vi "AssertControlValueByPath.vi"(0 "VI Reference In":refnum<vi>, 5 "Control Path":string[](array[string]), 11 "error in":errorcluster) -> (4 "VI Reference Out":refnum<vi>, 6 "Value":variant, 15 "error out":errorcluster)   [LabVIEW 2016]
doc: "This VI sets the value of top level controls in other VI"
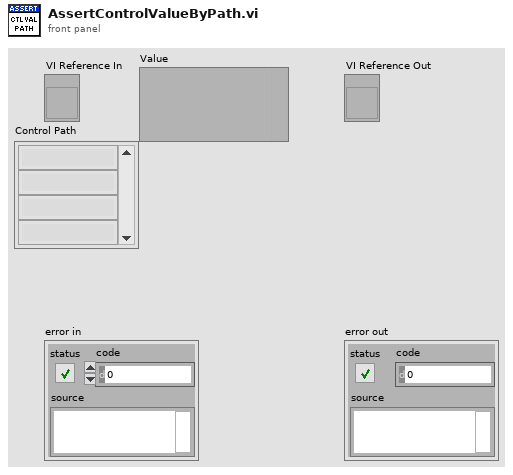
[diagram p1: front panel]
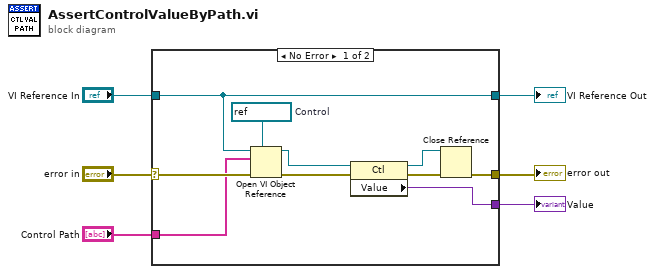
[diagram p0: block diagram]
diagram:
  n1 = case shown="No Error" "error in" {
    selector: "error in" -> [w15 w18]
    tunnel: "Control Path" -> [w14 _]
    tunnel: "VI Reference In" -> [w10 w17]
    tunnel: [w10 w17] -> w3
    tunnel: [w8 w18] -> w2
    tunnel: [w16 _] -> w1
    frame No Error {
      w12 = refnum<vi> refnum  # Control
      n2 = Open VI Object Reference(7:w12, 8:w15, 10:w14, 11:w10) -> (0:w11:errorcluster, 3:w13:refnum<vi>)
      n3 = property class="Ctl"(reference=w13, error in=w11) -> (reference out=w7:refnum<vi>, error out=w9:errorcluster, "Value"=w16:variant)
      n4 = Close Reference(reference=w7, error in (no error)=w9) -> (error out=w8:errorcluster)
    }
    frame Error {
    }
  }
  "error out" <- w2
  "VI Reference Out" <- w3
  "Value" <- w1
